vi "Selete_SW_Cmd2.vi"(1 "组合框":string(combo), 2 "H_32":bool[](array[boolean]), 3 "L_32":bool[](array[boolean]), 4 "64 SW OUT":bool[](array[boolean]), 5 "error in (no error)":errorcluster caption="错误输入（无错误）") -> (15 "OpenStr":string, 16 "ColseStr":string, 17 "OpenStr2":string, 19 "error out":errorcluster caption="错误输出")   [LabVIEW 2018]
panel:
  out "长度":i32
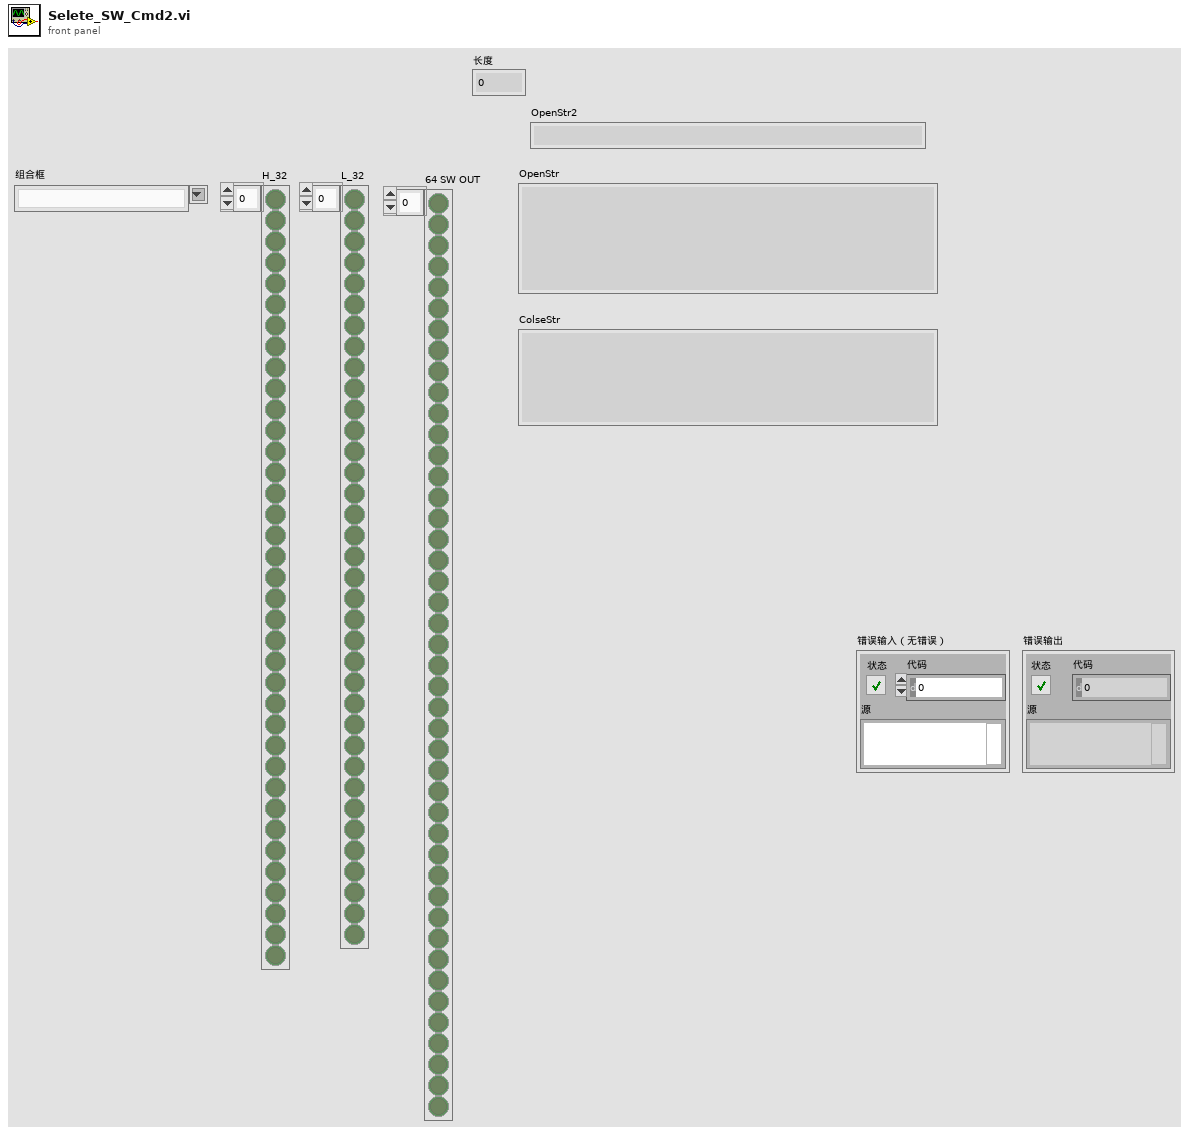
[diagram p1: front panel]
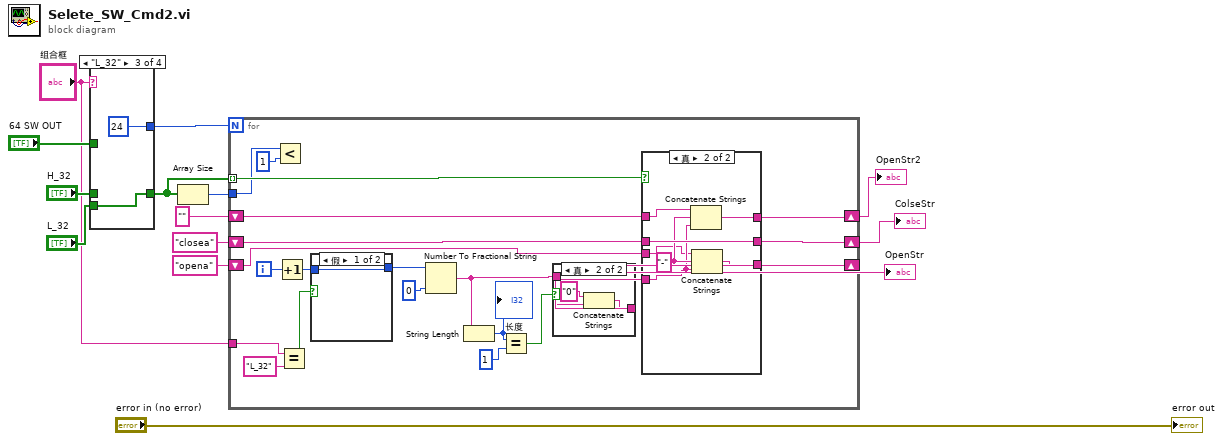
[diagram p0: block diagram]
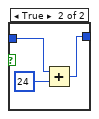
[diagram p2: hidden frame]
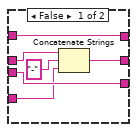
[diagram p4: hidden frame]
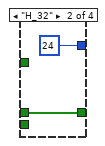
[diagram p6: hidden frame]
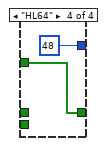
[diagram p7: hidden frame]
diagram:
  n1 = case shown="\"L_32\"" "组合框" {
    tunnel: "H_32" -> [_ w16 _ _]
    tunnel: "L_32" -> [_ _ w18 _]
    tunnel: "64 SW OUT" -> [_ _ _ w20]
    tunnel: [_ w16 w18 w20] -> w8
    tunnel: [_ 24 24 48] -> w11
    frame "假", Default {
    }
    frame "H_32" {
    }
    frame "L_32" {
    }
    frame "HL64" {
    }
  }
  n2 = Array Size(array=w8) -> (size(s)=w7:i32)
  n3 = for {
    N: w11 -> [_]
    tunnel: w8 -> [w38] mode=indexing
    shift-right: [w39] -> w6
    shift-left: "opena" -> [w37]
    shift-right: [w34] -> w5
    shift-left: "closea" -> [w36]
    tunnel: w7 -> [w33]
    tunnel: "组合框" -> [w24]
    shift-right: [w22] -> w1
    shift-left: "" -> [w21]
    i -> [w41]
    n4 = Less?(x=w33, y=1) -> ()  [unwired: 1 out]
    n5 = Increment(x=w41) -> (x+1=w26:i32)
    n6 = Equal?(x=w24, y="L_32") -> (x = y?=w23:bool)
    n7 = case shown="假" w23 {
      tunnel: w26 -> [w42 w45]
      tunnel: [w42 w44] -> w25
      frame False {
      }
      frame True {
        n8 = Add(x=w45, y=24) -> (x+y=w44:i32)
      }
    }
    n9 = Number To Fractional String(number=w25, precision (6)=i16 0 ("精度(6)")) -> (F-format string=w29:string)  [unwired: 2 in]
    n10 = String Length(string=w29) -> (length=w32:i32)
    "长度" <- w32
    n11 = Equal?(x=w32, y=1) -> (x = y?=w30:bool)
    n12 = case shown="真" w30 {
      tunnel: w29 -> [w46 w49]
      tunnel: [w46 w48] -> w28
      frame False {
      }
      frame True {
        n13 = Concatenate Strings("0" ("字符串"), w49) -> (w48:string)
      }
    }
    n14 = case shown="真" w38 {
      tunnel: w28 -> [w51 w59]
      tunnel: [w53 w62] -> w39
      tunnel: w37 -> [w53 w58]
      tunnel: w36 -> [w52 w61]
      tunnel: [w54 w61] -> w34
      tunnel: [w50 w57] -> w22
      tunnel: w21 -> [w50 w56]
      frame False {
        n15 = Concatenate Strings(w52, "-", w51) -> (w54:string)
      }
      frame True {
        w60 = "-"
        n16 = Concatenate Strings(w56, w60, w59) -> (w57:string)
        n17 = Concatenate Strings(w58, w60, w59) -> (w62:string)
      }
    }
  }
  "ColseStr" <- w5
  "OpenStr" <- w6
  "OpenStr2" <- w1
  "error out" <- "error in (no error)"
